vi "Comm_close 2d cdb waveform.vi"(8 "error in (no error)":errorcluster, 11 "WPL Comm (2D CDB) in":refnum<class "WPL Comm (2D CDB).lvclass">) -> (0 "error out":errorcluster)   [LabVIEW 2020, in "Internal Comm Classes.lvlib" / "WPL Comm (2D CDB).lvclass"]
uses:
  WPL Comm (2D CDB).lvclass
  D:/p4/penguin/lvaddon/Veristand/master/src/LabVIEW/vilib/NI VeriStand/Custom Device Waveform API/Internal Comm Classes/WPL Comm/WPL Comm.lvclass
  WPL Comm (2D CDB).lvclass/WPL Comm (2D CDB).ctl
  WPL Command.ctl
  WPL Comm.lvclass/WPL Comm.ctl
  Set ErrorQ on Variant.vi
  Send WPL Command.vi
  WPL Comm.lvclass
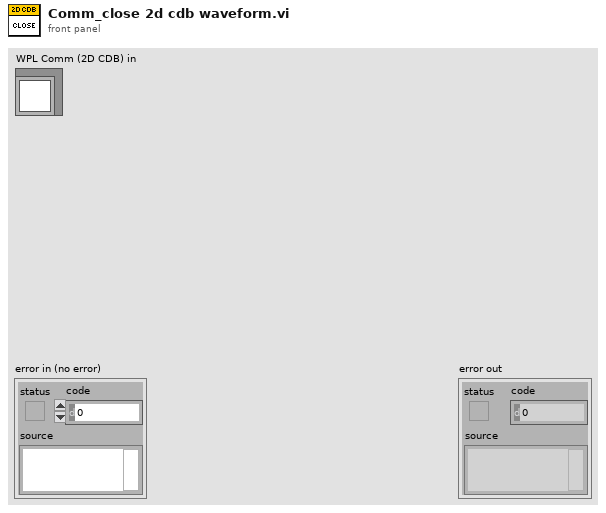
[diagram p1: front panel]
types:
  T1 = typedef "Internal Comm Classes.lvlib/WPL Comm.lvclass/WPL Command.ctl" = enum16{"Register 1D DBL Reader", "Unregister 1D DBL Reader", "Register 1D DBL Writer", "Register 2D DBL Writer", "Unregister 1D DBL Writer", "Unregister 2D DBL Writer", "DBL WFM Start", "WFM 1D DBL Data", "WFM 2D DBL Data", "Shut down", "Handle Error", "Register 1D CDB Reader", "Unregister 1D CDB Reader", "Register 1D CDB Writer", "Unregister 1D CDB Writer", "Register 2D CDB Writer", "Unregister 2D CDB Writer", "WFM 1D CDB Data", "WFM 2D CDB Data", "CDB WFM Start", "Error Shutdown", "Register Streams", "Unregister Streams", "Delete All Streams", "Get WFM DTs", "DBL WFM Multi Start", "CDB WFM Multi Start"}
  T2 = typedef "Internal Comm Classes.lvlib/WPL Comm (2D CDB).lvclass/Waveform 2d cdb queue.ctl" = refnum<queue>
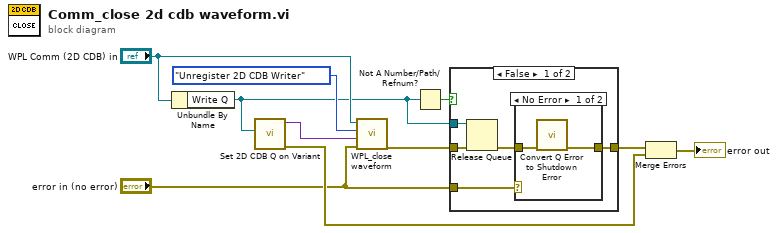
[diagram p0: block diagram]
diagram:
  n1 = Unbundle By Name("WPL Comm (2D CDB) in") -> ("Write Q"=w2:T2)
  n2 = call "Set 2D CDB Q on Variant.vi"("2D CDB Data Q"=w2) -> ("error out"=w10:errorcluster, "Variant out"=w6:variant)  [unwired: 8 in, 1 out]
  n3 = call "WPL_close waveform.vi"("error in (no error)"="error in (no error)", "Variant"=w6, "Command"=WPL_Command."Unregister 2D CDB Writer", "WPL Comm in"="WPL Comm (2D CDB) in") -> ("error out"=w5:errorcluster)  [unwired: 7 in]
  n4 = Not A Number/Path/Refnum?(number/path/refnum=w2) -> (NaN/Path/Refnum?=w1:bool)
  n5 = case shown="False" w1 {
    tunnel: w5 -> [w15 w19]
    tunnel: [w12 w19] -> w4
    tunnel: w2 -> [w14 _]
    tunnel: "error in (no error)" -> [w11 _]
    frame False {
      n6 = Release Queue(queue=w14, error in (no error)=w15) -> (error out=w13:errorcluster)  [unwired: 1 in, 2 out]
      n7 = case shown="No Error" w11 {
        tunnel: w13 -> [w17 w18]
        tunnel: [w16 w18] -> w12
        frame No Error {
          n8 = call "Convert Q Error to Shutdown Error.vi"("error in (no error)"=w17) -> ("error out"=w16:errorcluster)  [unwired: 10 in]
        }
        frame Error {
        }
      }
    }
    frame True {
    }
  }
  n9 = Merge Errors(w4, w10) -> (→"error out":errorcluster)
